vi "FTW-Supervisor-Launch.vi"(5 "FTW Supervisor Configuration":string="{\n  \"AppName\":         \"Your Application\",\n  \"AppVersionMajor\": 0,\n  \"AppVersionMinor\": 0,\n  \"AppVersionPatch\": 1,\n  \"Identity\":        \"FTW Application Supervisor\",\n  \"InboxAddress\":    \"tcp://127.0.0.1:38900\",\n  \"DashboardInboxAddress\":     \"ws://127.0.0.1:38901\",\n  \"DashboardPublisherAddress\": \"ws://127.0.0.1:38902\",\n  \"DashboardPageAddress\":      \"ws://127.0.0.1:38903\",\n  \"LogRetentionPolicy\": {\n    \"PersistToDisk\": true,\n    \"LogFilepath\": \"%LocalAppData%/Featherweight/FTWApplicationLog.db\",\n    \"MaxEventsToKeep\": 100000,\n    \"MaxActorsToRemember\": 1000\n  }\n}", 11 "error in":errorcluster) -> (4 "FTW Supervisor Connection":refnum<class "FTW-Supervisor-Connector.lvclass">, 6 "Supervisor Address":string, 15 "error out":errorcluster)   [LabVIEW 2014, in "FTW-Supervisor-Connector.lvclass"]
uses:
  connector/FTW-Supervisor-Connector.lvclass
  connector/FTW-Supervisor-Connector.lvclass/FTW-Supervisor-Connector.ctl
  FTW-Supervisor.lvclass
panel:
  # "Inputs"
  # "Outputs"
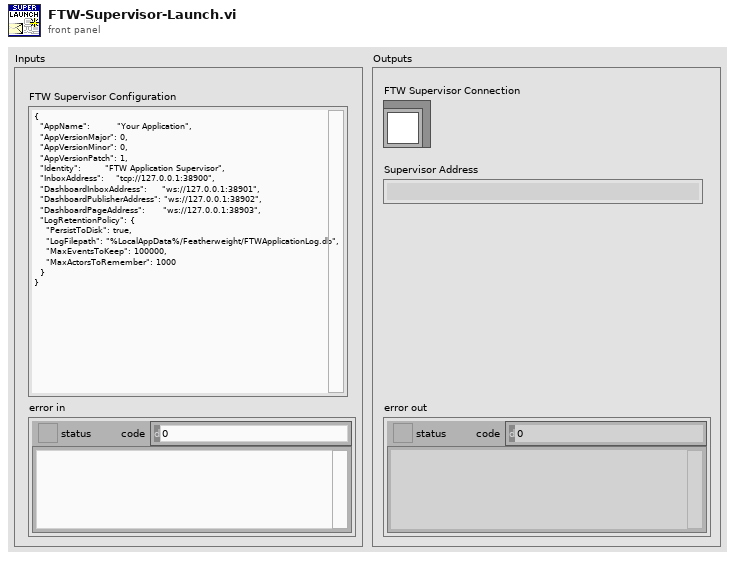
[diagram p1: front panel]
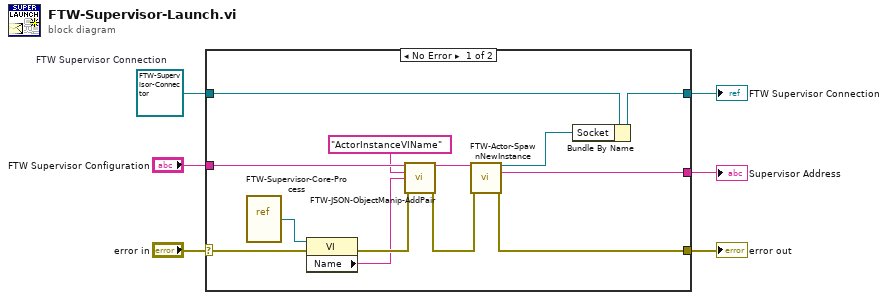
[diagram p0: block diagram]
diagram:
  w3 = refnum<class "FTW-Supervisor-Connector.lvclass"> refnum  # FTW Supervisor Connection
  n1 = case shown="No Error" "error in" {
    selector: "error in" -> [w17 w21]
    tunnel: [w19 w21] -> w6
    tunnel: [w8 w20] -> w4
    tunnel: w3 -> [w9 w20]
    tunnel: "FTW Supervisor Configuration" -> [w16 _]
    tunnel: [w10 _] -> w1
    frame No Error {
      n2 = vi-ref "FTW-Supervisor-Core-Process.vi"() -> (w18:refnum<vi>)
      n3 = property class="VI"(reference=w18, error in=w17) -> (error out=w15:errorcluster, "Name"=w12:string)  [unwired: 1 out]
      n4 = call "FTW-JSON-ObjectManip-AddPair.vi"("Input JSON Object"=w16, "Key"="ActorInstanceVIName", "Value"=w12, "error in"=w15) -> ("Output JSON Object"=w11:string, "error out"=w14:errorcluster)  [unwired: 10 in]
      n5 = call "FTW-Actor-SpawnNewInstance.vi"("Instance Configuration"=w11, "error in"=w14) -> ("FTW Actor Connector"=w7:refnum<data-value>, "Instance Inbox Address"=w10:string, "error out"=w19:errorcluster)  [unwired: 10 in, 1 out]
      n6 = Bundle By Name(cluster=w9, "Socket"=w7) -> (w8:refnum<class "FTW-Supervisor-Connector.lvclass">)
    }
    frame Error {
    }
  }
  "error out" <- w6
  "FTW Supervisor Connection" <- w4
  "Supervisor Address" <- w1
